vi "Test Git.vi"() -> ()   [LabVIEW 2019, in "Git.lvclass"]
uses:
  Git.lvclass
  Git.lvclass/Git.ctl
  <vilib>/LabVIEW Open Source Project/Unicity/RandomStringGenerator/RandomStringGenerator.lvclass
panel:
  out "String":string
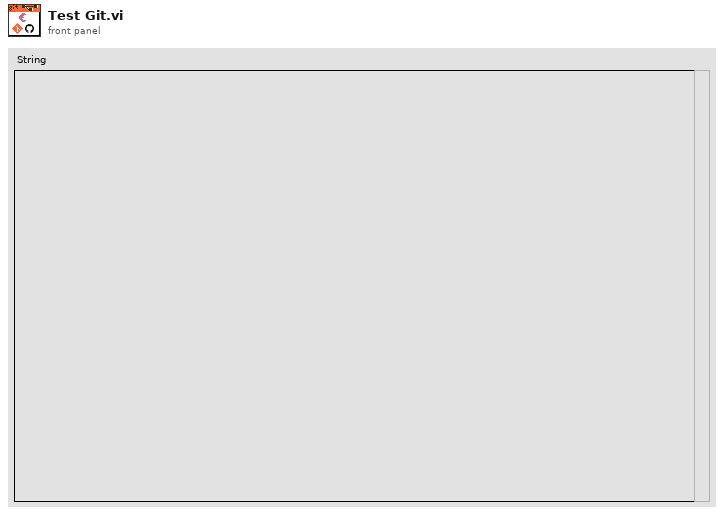
[diagram p1: front panel]
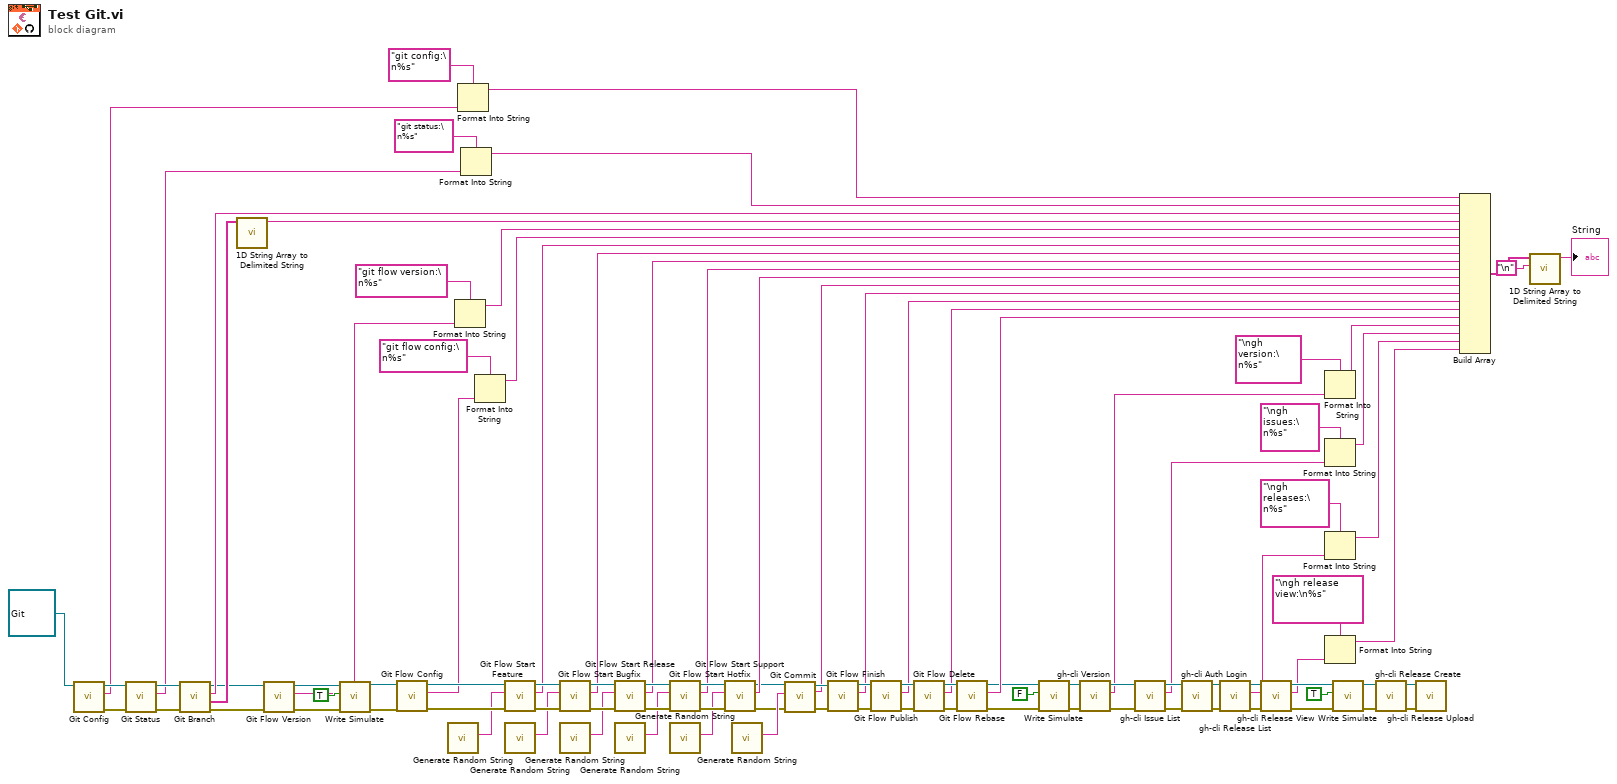
[diagram p0: block diagram]
diagram:
  n1 = call "Git Config.vi"("Git in"=refnum<class "Git.lvclass"> refnum) -> ("error out"=w61:errorcluster, "standard output"=w35:string, "Git out"=w62:refnum<class "Git.lvclass">)  [unwired: 8 in]
  n2 = call "Git Status.vi"("error in (no error)"=w61, "Git in"=w62) -> ("error out"=w60:errorcluster, "standard output"=w32:string, "Git out"=w64:refnum<class "Git.lvclass">)  [unwired: 7 in]
  n3 = call "Git Branch.vi"("error in (no error)"=w60, "Git in"=w64) -> ("error out"=w57:errorcluster, "all branches"=w63:string[], "active branch"=w59:string, "Git out"=w58:refnum<class "Git.lvclass">)  [unwired: 6 in]
  n4 = call <vilib>:"1D String Array to Delimited String.vi"("string array"=w63) -> ("delimited string"=w54:string)  [unwired: 10 in]
  n5 = call "Git Flow Version.vi"("error in (no error)"=w57, "Git in"=w58) -> ("error out"=w56:errorcluster, "version"=w29:string, "Git out"=w55:refnum<class "Git.lvclass">)  [unwired: 7 in]
  n6 = call "Write Simulate.vi"("error in (no error)"=w56, "Simulate"=TRUE, "Git in"=w55) -> ("error out"=w43:errorcluster, "Git out"=w42:refnum<class "Git.lvclass">)  [unwired: 7 in]
  n7 = call "Git Flow Config.vi"("error in (no error)"=w43, "Git in"=w42) -> ("error out"=w78:errorcluster, "standard output"=w26:string, "Git out"=w79:refnum<class "Git.lvclass">)  [unwired: 7 in]
  n8 = call <vilib>:"Generate Random String.vi"() -> ("Random String"=w28:string)  [unwired: 11 in]
  n9 = Format Into String(format string="git flow version:\n%s", w29) -> (resulting string=w3:string)  [unwired: 2 in, 1 out]
  n10 = Format Into String(format string="git config:\n%s", w35) -> (resulting string=w34:string)  [unwired: 2 in, 1 out]
  n11 = Format Into String(format string="git status:\n%s", w32) -> (resulting string=w31:string)  [unwired: 2 in, 1 out]
  n12 = Format Into String(format string="git flow config:\n%s", w26) -> (resulting string=w25:string)  [unwired: 2 in, 1 out]
  n13 = call "Git Flow Start Feature.vi"("error in (no error)"=w78, "name"=w28, "Git in"=w79) -> ("error out"=w96:errorcluster, "standard output"=w77:string, "Git out"=w97:refnum<class "Git.lvclass">)  [unwired: 6 in]
  n14 = call <vilib>:"Generate Random String.vi"() -> ("Random String"=w83:string)  [unwired: 11 in]
  n15 = call "Git Flow Start Bugfix.vi"("error in (no error)"=w96, "name"=w83, "Git in"=w97) -> ("error out"=w94:errorcluster, "standard output"=w76:string, "Git out"=w95:refnum<class "Git.lvclass">)  [unwired: 6 in]
  n16 = call <vilib>:"Generate Random String.vi"() -> ("Random String"=w82:string)  [unwired: 11 in]
  n17 = call "Git Flow Start Release.vi"("error in (no error)"=w94, "version"=w82, "Git in"=w95) -> ("error out"=w92:errorcluster, "standard output"=w75:string, "Git out"=w93:refnum<class "Git.lvclass">)  [unwired: 6 in]
  n18 = call <vilib>:"Generate Random String.vi"() -> ("Random String"=w81:string)  [unwired: 11 in]
  n19 = call "Git Flow Start Hotfix.vi"("error in (no error)"=w92, "version"=w81, "Git in"=w93) -> ("error out"=w90:errorcluster, "standard output"=w74:string, "Git out"=w91:refnum<class "Git.lvclass">)  [unwired: 6 in]
  n20 = call <vilib>:"Generate Random String.vi"() -> ("Random String"=w80:string)  [unwired: 11 in]
  n21 = call "Git Flow Start Support.vi"("error in (no error)"=w90, "version"=w80, "Git in"=w91) -> ("error out"=w41:errorcluster, "standard output"=w73:string, "Git out"=w40:refnum<class "Git.lvclass">)  [unwired: 6 in]
  n22 = call <vilib>:"Generate Random String.vi"() -> ("Random String"=w65:string)  [unwired: 11 in]
  n23 = call "Git Commit.vi"("error in (no error)"=w41, "Commit Message"=w65, "Git in"=w40) -> ("error out"=w38:errorcluster, "standard output"=w37:string, "Git out"=w39:refnum<class "Git.lvclass">)  [unwired: 6 in]
  n24 = call "Git Flow Finish.vi"("error in (no error)"=w38, "Git in"=w39) -> ("error out"=w88:errorcluster, "standard output"=w72:string, "Git out"=w89:refnum<class "Git.lvclass">)  [unwired: 7 in]
  n25 = call "Git Flow Publish.vi"("error in (no error)"=w88, "Git in"=w89) -> ("error out"=w86:errorcluster, "standard output"=w71:string, "Git out"=w87:refnum<class "Git.lvclass">)  [unwired: 7 in]
  n26 = call "Git Flow Delete.vi"("error in (no error)"=w86, "Git in"=w87) -> ("error out"=w84:errorcluster, "standard output"=w70:string, "Git out"=w85:refnum<class "Git.lvclass">)  [unwired: 7 in]
  n27 = call "Git Flow Rebase.vi"("error in (no error)"=w84, "Git in"=w85) -> ("error out"=w47:errorcluster, "standard output"=w69:string, "Git out"=w46:refnum<class "Git.lvclass">)  [unwired: 7 in]
  n28 = call "Write Simulate.vi"("error in (no error)"=w47, "Simulate"=FALSE, "Git in"=w46) -> ("error out"=w44:errorcluster, "Git out"=w45:refnum<class "Git.lvclass">)  [unwired: 7 in]
  n29 = call "gh-cli Version.vi"("error in (no error)"=w44, "Git in"=w45) -> ("error out"=w51:errorcluster, "version"=w23:string, "Git out"=w52:refnum<class "Git.lvclass">)  [unwired: 7 in]
  n30 = call "gh-cli Issue List.vi"("error in (no error)"=w51, "Git in"=w52) -> ("error out"=w49:errorcluster, "Issues"=w1:string, "Git out"=w50:refnum<class "Git.lvclass">)  [unwired: 7 in]
  n31 = call "gh-cli Auth Login.vi"("error in (no error)"=w49, "Git in"=w50) -> ("error out"=w20:errorcluster, "Git out"=w21:refnum<class "Git.lvclass">)  [unwired: 8 in]
  n32 = call "gh-cli Release List.vi"("error in (no error)"=w20, "Git in"=w21) -> ("error out"=w18:errorcluster, "Release(s)"=w7:string, "Git out"=w19:refnum<class "Git.lvclass">)  [unwired: 7 in]
  n33 = call "gh-cli Release View.vi"("error in (no error)"=w18, "Git in"=w19) -> ("error out"=w14:errorcluster, "standard output"=w5:string, "Git out"=w13:refnum<class "Git.lvclass">)  [unwired: 7 in]
  n34 = Format Into String(format string="\ngh version:\n%s", w23) -> (resulting string=w22:string)  [unwired: 2 in, 1 out]
  n35 = Format Into String(format string="\ngh issues:\n%s", w1) -> (resulting string=w9:string)  [unwired: 2 in, 1 out]
  n36 = Format Into String(format string="\ngh releases:\n%s", w7) -> (resulting string=w2:string)  [unwired: 2 in, 1 out]
  n37 = Format Into String(format string="\ngh release view:\n%s", w5) -> (resulting string=w4:string)  [unwired: 2 in, 1 out]
  n38 = call "Write Simulate.vi"("error in (no error)"=w14, "Simulate"=TRUE, "Git in"=w13) -> ("error out"=w12:errorcluster, "Git out"=w11:refnum<class "Git.lvclass">)  [unwired: 7 in]
  n39 = call "gh-cli Release Create.vi"("error in (no error)"=w12, "Git in"=w11) -> ("error out"=w16:errorcluster, "Git out"=w17:refnum<class "Git.lvclass">)  [unwired: 7 in, 1 out]
  n40 = call "gh-cli Release Upload.vi"("error in (no error)"=w16, "Git in"=w17) -> ()  [unwired: 7 in, 3 out]
  n41 = Build Array(w34, w31, w59, w54, w3, w25, w77, w76, w75, w74, w73, w37, w72, w71, w70, w69, w22, w9, w2, w4) -> (w68:string[])
  n42 = call <vilib>:"1D String Array to Delimited String.vi"("delimiter"="\n", "string array"=w68) -> ("delimited string"=→"String":string)  [unwired: 9 in]
